vi "Intake And Elevator Loop.vi"(7 "Climbing?":bool) -> (3 "Intake Left Power":dbl, 4 "Intake Right Power":dbl, 6 "Intake Open":bool, 8 "Shift?":bool, 10 "Intake Angle":dbl, 15 "Elevator Power":dbl)   [LabVIEW 2017]
uses:
  Common Code/Intake And Elevator States.ctl
  Robot Global Data.vi
  <vilib>/addons/control/pid/pid.llb/PID (DBL).vi
  <vilib>/addons/control/pid/NI_PID_pid.lvlib
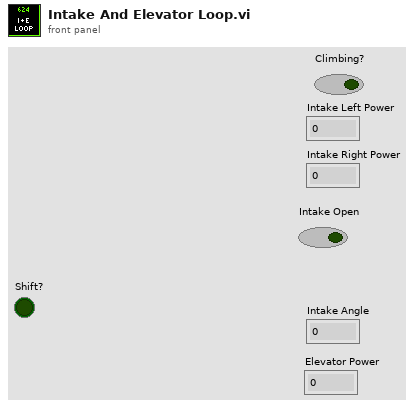
[diagram p1: front panel]
types:
  T1 = typedef "Intake And Elevator States.ctl" = enum16{"Reset", "Shoot Cube", "Drop Cube", "Idle", "Pick Up Cube", "Switch", "Scale ", "Endgame"}
  T2 = typedef "Intake And Elevator Command Cluster.ctl" = cluster{"States ":T1, "Grab?":bool, "Drop?":bool, "Mode":T3, "Override Lift":bool, "Override Lift":dbl, "High?":bool, "Override Angle":bool, "Override Angle":dbl}
  T3 = typedef "Intake and Elevator Mode.ctl" = enum16{"Auto", "Not Auto"}
  T4 = typedef "Dashboard Control Data.ctl" = cluster{"Drivetrain Settings Cluster":T5, "Intake Presets":T8, "Elevator Settings Cluster":T9, "Drivetrain Encoder Values":T11, "Auton Chooser":T12, "Auton Presets":cluster{"Start Position":dbl}, "Elevator Encoder Values":T13, "Pressure M":dbl, "Pressure B":dbl, "Zero All?":bool, "Enable Vision":bool}
  T5 = typedef "Drivetrain Settings Cluster.ctl" = cluster{"Gyro Steer PID Gains":T6, "Distance Drive PID Gains":T6, "Drive Tolerance":dbl, "Gyro Tolerance":dbl, "Gyro Output":dbl, "Distance Output":dbl, "Y Power Multiplier":dbl, "Turn Power Multiplier":dbl, "Creep Rate":dbl, "Encoder Reset":bool, "DT Mode Modifier":enum16{"None, Default", "Cube", "Square"}, "Left Encoder Tick Constant":dbl, "Right Encoder Tick Constant":dbl, "Shift Speed":dbl, "Zero Gyro":bool, "Y min":dbl, "Y max":dbl, "X min":dbl, "X max":dbl, "Finish Velocity":dbl, "Anti-Tip Settings":T7}
  T6 = typedef "PID Gains Cluster.ctl" = cluster{"Proportional Gain":dbl, "Integral Time":dbl, "Derivative Time":dbl}
  T7 = typedef "Anti-Tip Settings.ctl" = cluster{"Pitch Tip Constant":dbl, "Wheel Diameter":dbl, "Gearbox Reduction":dbl, "Motor Count":dbl, "Mass of Robot":dbl, "Almost Tip Constant":dbl, "Dist to CG":dbl}
  T8 = typedef "Intake Presets.ctl" = cluster{"Idle Angle":dbl, "Mid Angle":dbl, "Low Angle":dbl, "Outtake Power":dbl, "Intake Power":dbl, "Unstuck":dbl, "Angle Tolerance":dbl, "Max Angle":dbl, "Max Current":dbl, "Current Trip Time":dbl, "Reset Encoder?":bool, "Encoder Scale":dbl, "PID gains":cluster{"proportional gain (Kc)":dbl, "integral time (Ti, min)":dbl, "derivative time (Td, min)":dbl}, "output range":cluster{"output high":dbl, "output low":dbl}, "IR Constant Pull Rate":dbl, "Shoot Angle":dbl}
  T9 = typedef "Elevator Settings Cluster.ctl" = cluster{"Ground Height":dbl, "Switch Height":dbl, "Scale High Height ":dbl, "Scale Low Height":dbl, "Elevator PID Gains":T10, "Elevator Tolerance":dbl, "Reset Encoders":bool, "Encoder Scale":dbl, "Max Height":dbl, "Mid Height":dbl, "output range":cluster{"output high":dbl, "output low":dbl}, "Upper Slow Down Tolerance":dbl, "Tick Constant":dbl, "Tip Constant":dbl, "Slow Down Multiplier":dbl, "Almost Tip Constant":dbl, "Bottom Trip Offset":dbl, "Lower Slow Down Tolerance":dbl}
  T10 = typedef "PID Gains.ctl" = cluster{"proportional gain (Kc)":dbl, "integral time (Ti, min)":dbl, "derivative time (Td, min)":dbl}
  T11 = typedef "DT Encoder Values.ctl" = cluster{"Left Encoder":cluster{"Distance":dbl, "Speed":dbl, "Tick":dbl}, "Right Encoder":cluster{"Distance":dbl, "Speed":dbl, "Tick":dbl}}
  T12 = typedef "Auton Chooser.ctl" = cluster{"Left":bool, "Center":bool, "Right":bool, "Scale":bool, "Both":bool, "Switch":bool, "Test":bool, "No Script":bool, "Drive PID":bool, "Elevator PID":bool, "Gyro PID":bool}
  T13 = typedef "Elevator Encoder Values.ctl" = cluster{"Encoder Values":cluster{"Distance":dbl, "Speed":dbl, "Tick":dbl}}
  T14 = typedef "Elevator Status Cluster.ctl" = cluster{"Finished":bool, "Elevator Power":dbl, "Elevator State":T15, "Elevator Mode":T16, "Elevator Height":dbl, "At Bottom?":bool, "At Top?":bool, "Scale high?":bool, "PID Output":dbl, "2nd Gear":bool}
  T15 = typedef "Elevator State.ctl" = enum16{"Idle", "Ground", "Mid", "Scale", "Switch"}
  T16 = typedef "Elevator Mode.ctl" = enum16{"Semi Auto", "Manual", "Auto"}
  T17 = typedef "Intake Status Cluster.ctl" = cluster{"Intake Mode":T18, "Intake States":T19, "Intake Current Angle":dbl, "Cube In Posession?":bool, "Intake Wrist Up?":bool, "Right Roller Power":dbl, "Angle Power":dbl, "Left Roller Power":dbl}
  T18 = typedef "Intake Mode.ctl" = enum16{"Auto", "Semi Auto", "Manual"}
  T19 = typedef "Intake States.ctl" = enum16{"Zero", "Override Angle", "Idle", "Drop Mid", "Drop Low", "Outtake", "Intake"}
  T20 = cluster{"proportional gain (Kc)":dbl, "integral time (Ti, min)":dbl, "derivative time (Td, min)":dbl}
  T21 = typedef "Robot Info.ctl" = cluster{"FMS":bool, "Switch and Scale Sides":string, "Event Name":string, "Alliance":T22, "Position":T23, "Match Number":u16, "Robot Mode":T24, "Match Time(s)":sgl}
  T22 = typedef "WPI_DriverStationAllianceInfo.ctl" = enum16{"Red", "Blue", "Invalid"}
  T23 = typedef "WPI_DriverStationPositionInfo.ctl" = enum16{"1", "2", "3"}
  T24 = typedef "WPI_DriverStationRobotMode2.ctl" = enum16{"Autonomous Disabled", "Autonomous Enabled", "Teleop Disabled", "Teleop Enabled", "Disconnected", "Finish", "Test Disabled", "Test Enabled", "Emergency Stopped"}
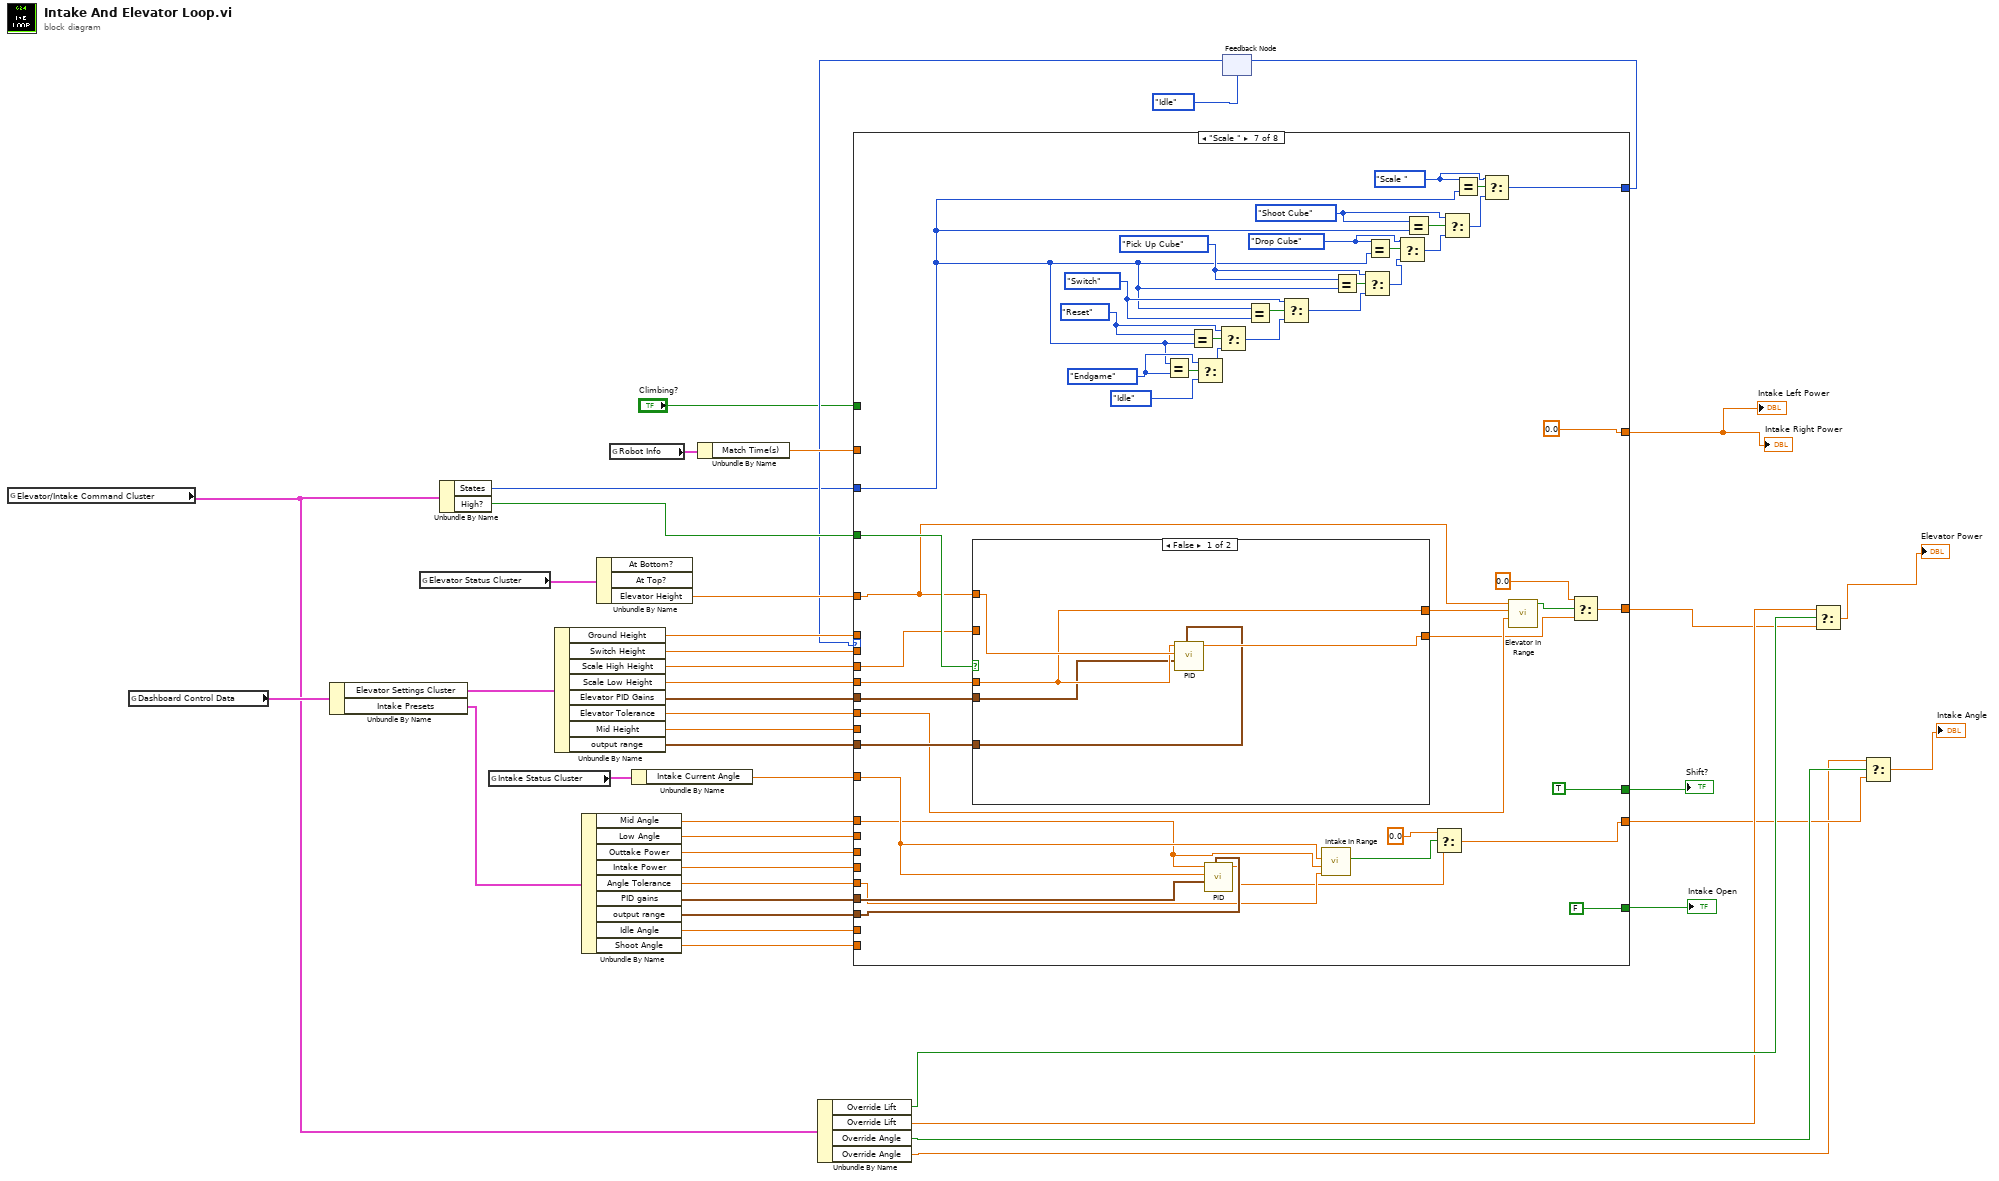
[diagram p0: block diagram]
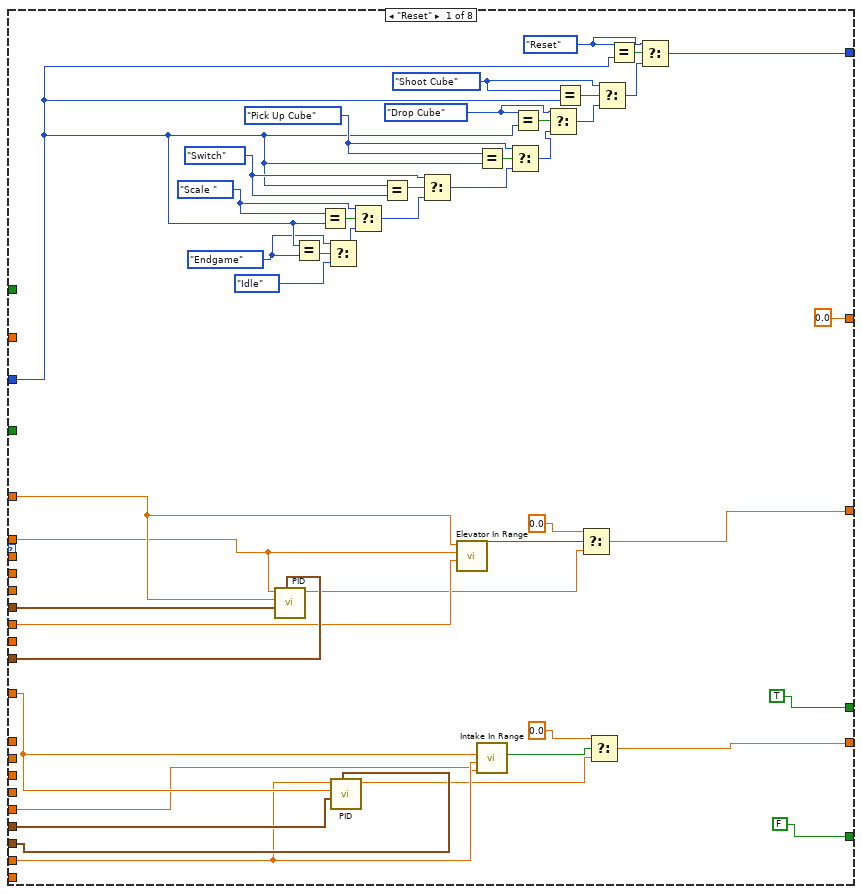
[diagram p2: hidden frame]
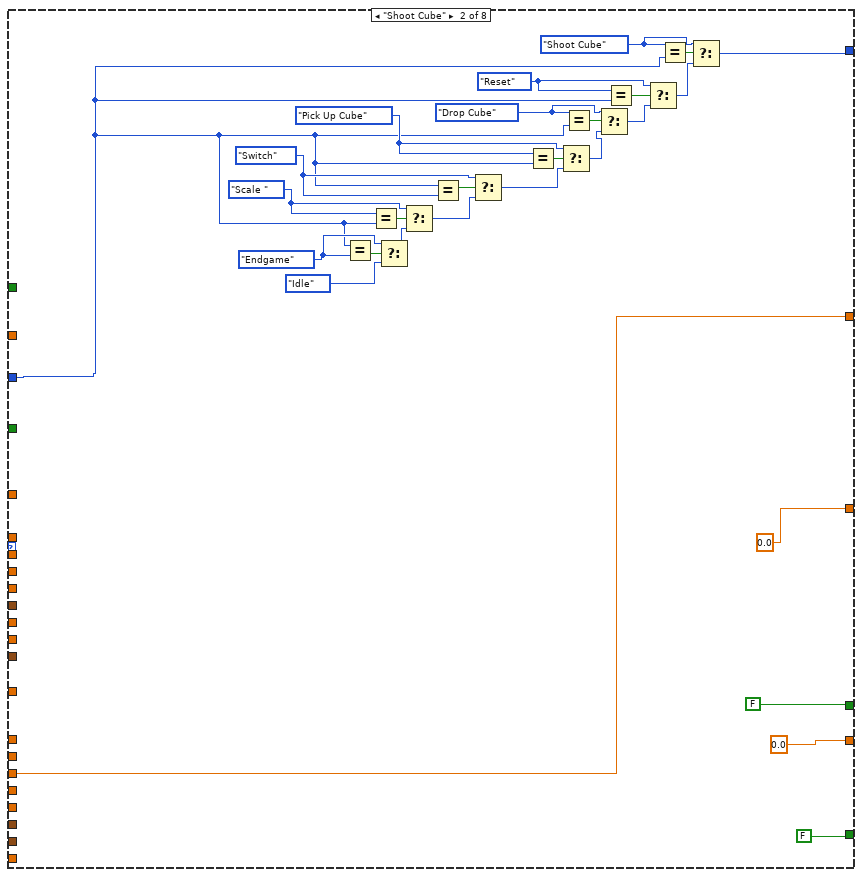
[diagram p3: hidden frame]
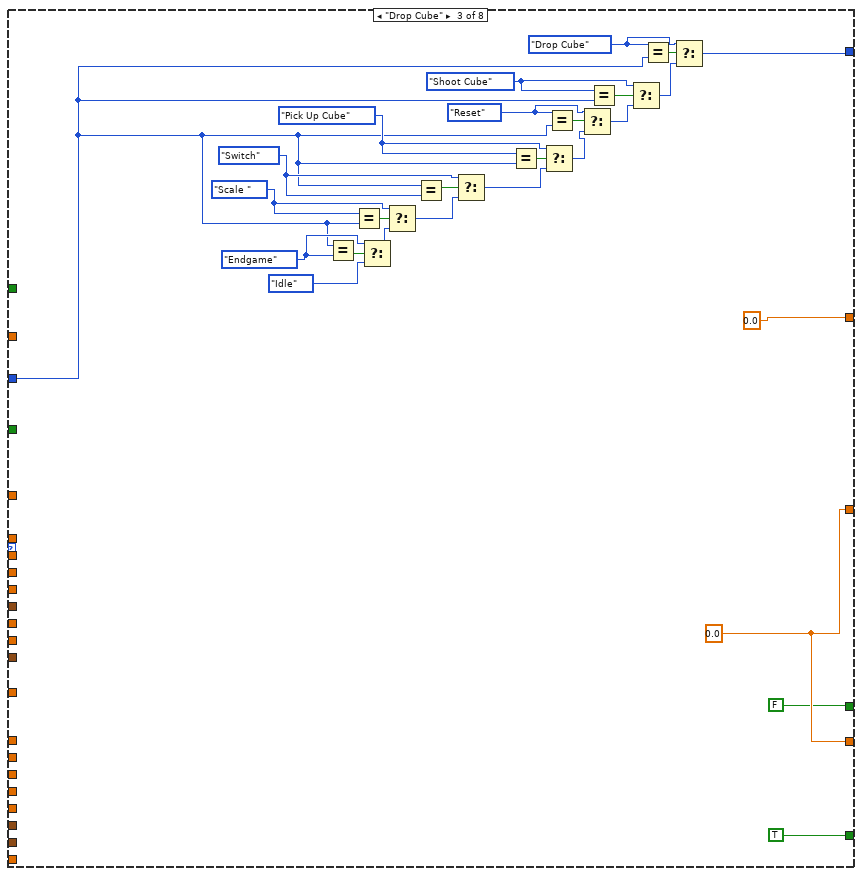
[diagram p4: hidden frame]
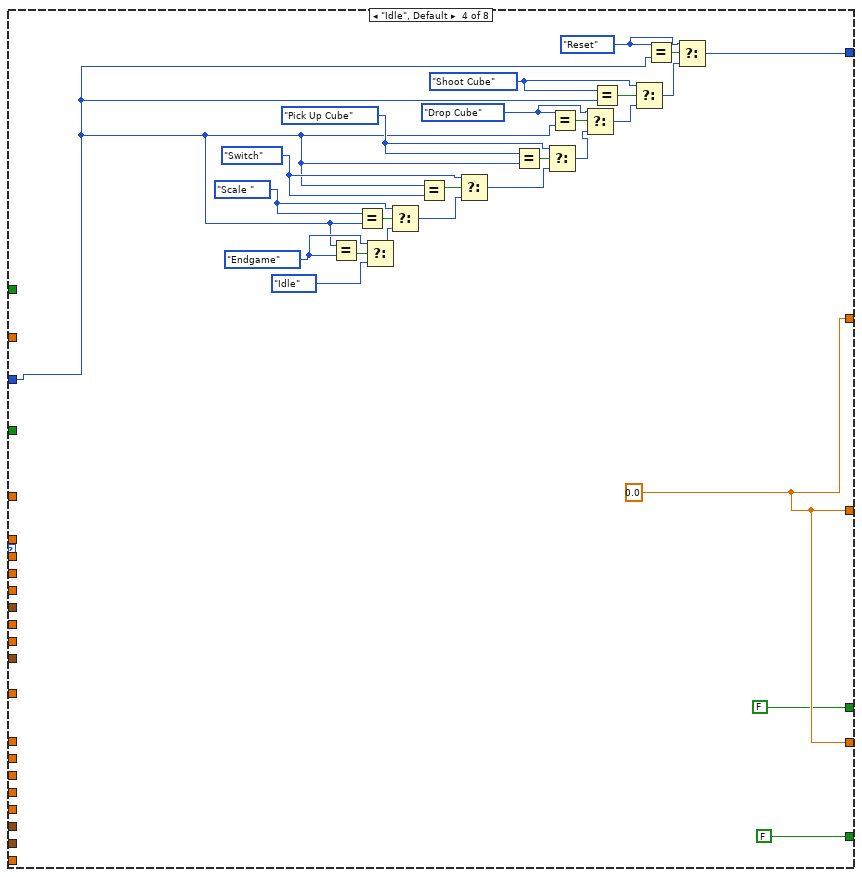
[diagram p5: hidden frame]
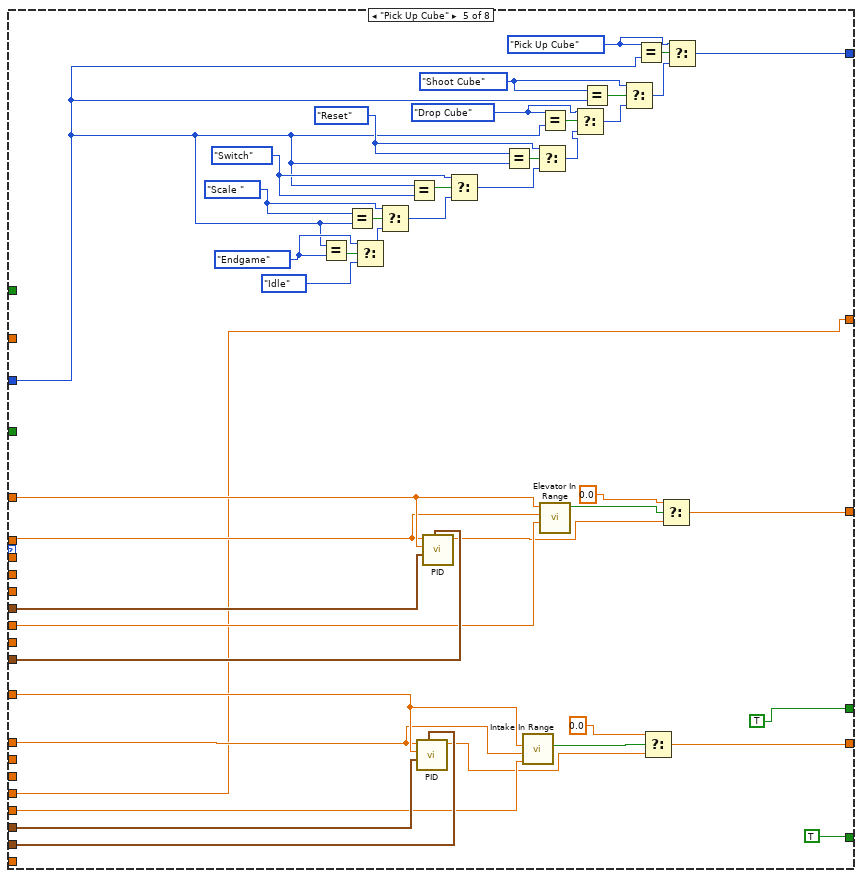
[diagram p6: hidden frame]
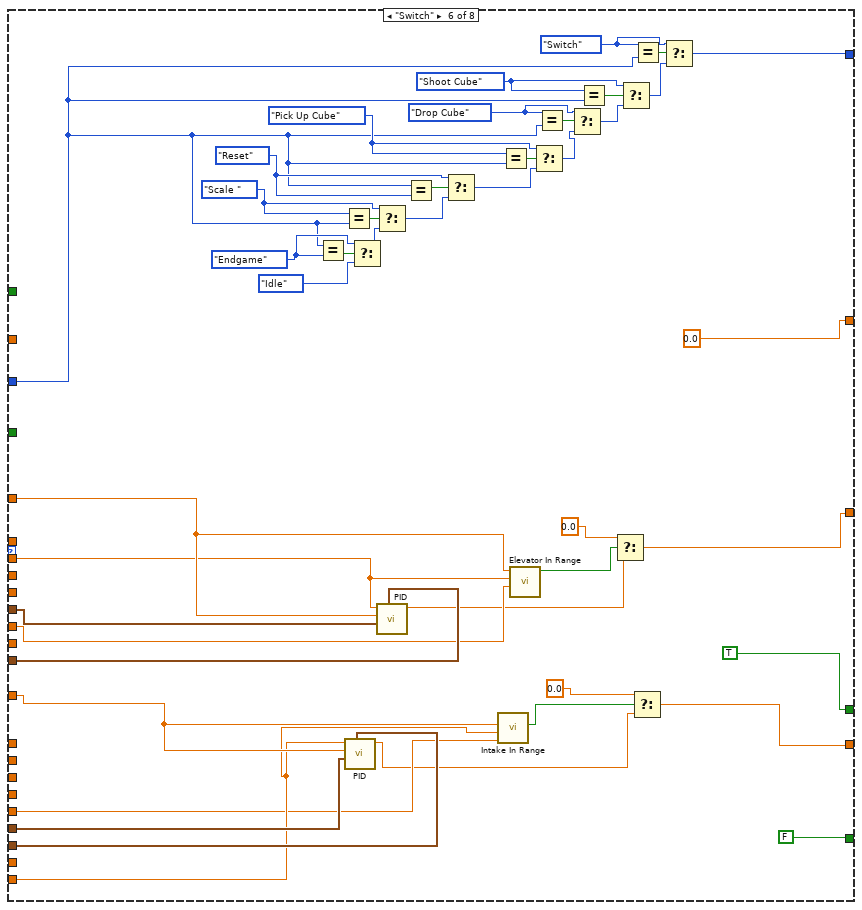
[diagram p7: hidden frame]
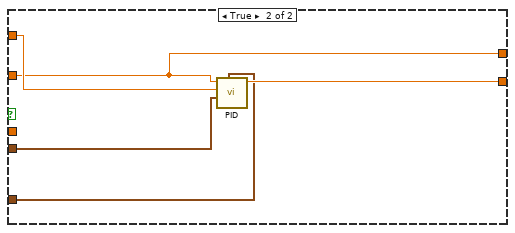
[diagram p8: hidden frame]
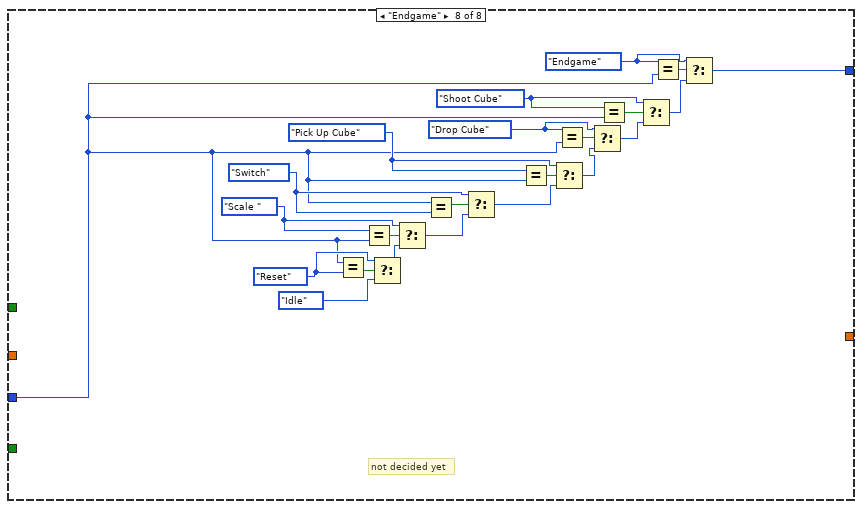
[diagram p9: hidden frame]
diagram:
  n1 = global read "Robot Global Data.vi" "Elevator/Intake Command Cluster"() -> (w9:T2)
  n2 = global read "Robot Global Data.vi" "Dashboard Control Data"() -> (w44:T4)
  n3 = Unbundle By Name(w44) -> ("Elevator Settings Cluster"=w43:T9, "Intake Presets"=w42:T8)
  n4 = global read "Robot Global Data.vi" "Elevator Status Cluster"() -> (w41:T14)
  n5 = Unbundle By Name(w9) -> ("States"=w12:T1, "High?"=w27:bool)
  n6 = global read "Robot Global Data.vi" "Intake Status Cluster"() -> (w40:T17)
  n7 = Unbundle By Name(w43) -> ("Ground Height"=w34:dbl, "Switch Height"=w28:dbl, "Scale High Height"=w26:dbl, "Scale Low Height"=w25:dbl, "Elevator PID Gains"=w32:T10, "Elevator Tolerance"=w30:dbl, "Mid Height"=w14:dbl, "output range"=w31:cluster{"output high":dbl, "output low":dbl})
  n8 = Unbundle By Name(w42) -> ("Mid Angle"=w29:dbl, "Low Angle"=w18:dbl, "Outtake Power"=w21:dbl, "Intake Power"=w19:dbl, "Angle Tolerance"=w37:dbl, "PID gains"=w35:T20, "output range"=w36:cluster{"output high":dbl, "output low":dbl}, "Idle Angle"=w39:dbl, "Shoot Angle"=w15:dbl)
  n9 = Unbundle By Name(w41) -> ("Elevator Height"=w33:dbl)  [unwired: 2 out]
  n10 = global read "Robot Global Data.vi" "Robot Info"() -> (w24:T21)
  n11 = Unbundle By Name(w40) -> ("Intake Current Angle"=w38:dbl)
  n12 = Unbundle By Name(w24) -> ("Match Time(s)"=w23:sgl)
  n13 = Unbundle By Name(w9) -> ("Override Lift"=w8:bool, "Override Lift"=w7:dbl, "Override Angle"=w4:bool, "Override Angle"=w1:dbl)
  n14 = feedback #1(Intake_And_Elevator_States."Idle" ("States")) -> (w13:T1)
  n15 = case shown="\"Scale \"" w13 {
    tunnel: w39 -> [w76 _ _ _ _ _ _ _]
    tunnel: w38 -> [w77 _ _ _ w203 w253 w290 _]
    tunnel: w37 -> [w75 _ _ _ w201 w251 w288 _]
    tunnel: w36 -> [w78 _ _ _ w212 w255 w291 _]
    tunnel: w35 -> [w79 _ _ _ w213 w254 w292 _]
    tunnel: w34 -> [w85 _ _ _ w208 _ _ _]
    tunnel: w33 -> [w86 _ _ _ w209 w246 w295 _]
    tunnel: w32 -> [w88 _ _ _ w211 w257 w301 _]
    tunnel: w31 -> [w87 _ _ _ w210 w256 w300 _]
    tunnel: w30 -> [w84 _ _ _ w207 w244 w297 _]
    tunnel: w29 -> [_ _ _ _ w202 _ w289 _]
    tunnel: w28 -> [_ _ _ _ _ w245 _ _]
    tunnel: w27 -> [_ _ _ _ _ _ w304 _]
    tunnel: w26 -> [_ _ _ _ _ _ w303 _]
    tunnel: w25 -> [_ _ _ _ _ _ w302 _]
    tunnel: w23 -> [_ _ _ _ _ _ _ _]
    tunnel: [w80 0.0 w142 w169 w197 w240 w299 _] -> w6
    tunnel: [w71 0.0 w142 w169 w196 w247 w284 _] -> w2
    tunnel: w21 -> [_ w114 _ _ _ _ _ _]
    tunnel: [0.0 w114 0.0 w169 w193 0.0 0.0 _] -> w20
    tunnel: w19 -> [_ _ _ _ w193 _ _ _]
    tunnel: w18 -> [_ _ _ _ _ _ _ _]
    tunnel: [FALSE FALSE TRUE FALSE TRUE FALSE FALSE _] -> w17
    tunnel: [TRUE FALSE FALSE FALSE TRUE TRUE TRUE _] -> w16
    tunnel: w15 -> [_ _ _ _ _ w252 _ _]
    tunnel: w14 -> [_ _ _ _ _ _ _ _]
    tunnel: w12 -> [w50 w90 w118 w145 w171 w215 w259 w316]
    tunnel: [w45 w89 w117 w144 w170 w214 w258 w315] -> w11
    tunnel: "Climbing?" -> [_ _ _ _ _ _ _ _]
    frame "Reset" {
      w48 = Intake_And_Elevator_States."Endgame" ("States")
      w52 = Intake_And_Elevator_States."Scale " ("States")
      w56 = Intake_And_Elevator_States."Switch" ("States")
      w58 = Intake_And_Elevator_States."Pick Up Cube" ("States")
      w61 = Intake_And_Elevator_States."Drop Cube" ("States")
      w64 = Intake_And_Elevator_States."Shoot Cube" ("States")
      w66 = Intake_And_Elevator_States."Reset" ("States")
      n16 = call-poly <vilib>:"PID.vi"("output range"=w87, "PID gains"=w88, "process variable"=w86, "setpoint"=w85) -> ("output"=w81:dbl)  [unwired: 6 in, 1 out]
      n17 = Equal?(x=w50, y=w48) -> (x = y?=w49:bool)
      n18 = Equal?(x=w52, y=w50) -> (x = y?=w53:bool)
      n19 = Select(t=w48, s=w49, f=Intake_And_Elevator_States."Idle" ("States")) -> (s? t:f=w47:T1)
      n20 = call-poly <vilib>:"PID.vi"("output range"=w78, "PID gains"=w79, "process variable"=w77, "setpoint"=w76) -> ("output"=w72:dbl)  [unwired: 6 in, 1 out]
      n21 = Select(t=w52, s=w53, f=w47) -> (s? t:f=w51:T1)
      n22 = Equal?(x=w50, y=w56) -> (x = y?=w57:bool)
      n23 = Select(t=w56, s=w57, f=w51) -> (s? t:f=w55:T1)
      n24 = call "Elevator In Range.vi"("Height Tolerance"=w84, "Target Height"=w85, "Actual Height"=w86) -> ("In Range"=w83:bool)  [unwired: 8 in]
      n25 = Equal?(x=w58, y=w50) -> (x = y?=w59:bool)
      n26 = call "Intake In Range.vi"("Angle Tolerance"=w75, "Target Height"=w76, "Actual Height"=w77) -> ("In Range?"=w74:bool)  [unwired: 8 in]
      n27 = Select(t=w58, s=w59, f=w55) -> (s? t:f=w54:T1)
      n28 = Equal?(x=w61, y=w50) -> (x = y?=w62:bool)
      n29 = Select(t=w61, s=w62, f=w54) -> (s? t:f=w60:T1)
      n30 = Equal?(x=w64, y=w50) -> (x = y?=w65:bool)
      n31 = Select(t=0.0, s=w83, f=w81) -> (s? t:f=w80:dbl)
      n32 = Select(t=0.0, s=w74, f=w72) -> (s? t:f=w71:dbl)
      n33 = Select(t=w64, s=w65, f=w60) -> (s? t:f=w63:T1)
      n34 = Equal?(x=w66, y=w50) -> (x = y?=w67:bool)
      n35 = Select(t=w66, s=w67, f=w63) -> (s? t:f=w45:T1)
    }
    frame "Shoot Cube" {
      w93 = Intake_And_Elevator_States."Endgame" ("States")
      w96 = Intake_And_Elevator_States."Scale " ("States")
      w100 = Intake_And_Elevator_States."Switch" ("States")
      w102 = Intake_And_Elevator_States."Pick Up Cube" ("States")
      w105 = Intake_And_Elevator_States."Drop Cube" ("States")
      w108 = Intake_And_Elevator_States."Reset" ("States")
      w110 = Intake_And_Elevator_States."Shoot Cube" ("States")
      n36 = Equal?(x=w90, y=w93) -> (x = y?=w94:bool)
      n37 = Equal?(x=w96, y=w90) -> (x = y?=w97:bool)
      n38 = Select(t=w93, s=w94, f=Intake_And_Elevator_States."Idle" ("States")) -> (s? t:f=w92:T1)
      n39 = Select(t=w96, s=w97, f=w92) -> (s? t:f=w95:T1)
      n40 = Equal?(x=w90, y=w100) -> (x = y?=w101:bool)
      n41 = Select(t=w100, s=w101, f=w95) -> (s? t:f=w99:T1)
      n42 = Equal?(x=w102, y=w90) -> (x = y?=w103:bool)
      n43 = Select(t=w102, s=w103, f=w99) -> (s? t:f=w98:T1)
      n44 = Equal?(x=w105, y=w90) -> (x = y?=w106:bool)
      n45 = Select(t=w105, s=w106, f=w98) -> (s? t:f=w104:T1)
      n46 = Equal?(x=w108, y=w90) -> (x = y?=w109:bool)
      n47 = Select(t=w108, s=w109, f=w104) -> (s? t:f=w107:T1)
      n48 = Equal?(x=w110, y=w90) -> (x = y?=w111:bool)
      n49 = Select(t=w110, s=w111, f=w107) -> (s? t:f=w89:T1)
    }
    frame "Drop Cube" {
      w121 = Intake_And_Elevator_States."Endgame" ("States")
      w124 = Intake_And_Elevator_States."Scale " ("States")
      w128 = Intake_And_Elevator_States."Switch" ("States")
      w130 = Intake_And_Elevator_States."Pick Up Cube" ("States")
      w133 = Intake_And_Elevator_States."Reset" ("States")
      w136 = Intake_And_Elevator_States."Shoot Cube" ("States")
      w138 = Intake_And_Elevator_States."Drop Cube" ("States")
      w142 = 0.0
      n50 = Equal?(x=w118, y=w121) -> (x = y?=w122:bool)
      n51 = Equal?(x=w124, y=w118) -> (x = y?=w125:bool)
      n52 = Select(t=w121, s=w122, f=Intake_And_Elevator_States."Idle" ("States")) -> (s? t:f=w120:T1)
      n53 = Select(t=w124, s=w125, f=w120) -> (s? t:f=w123:T1)
      n54 = Equal?(x=w118, y=w128) -> (x = y?=w129:bool)
      n55 = Select(t=w128, s=w129, f=w123) -> (s? t:f=w127:T1)
      n56 = Equal?(x=w130, y=w118) -> (x = y?=w131:bool)
      n57 = Select(t=w130, s=w131, f=w127) -> (s? t:f=w126:T1)
      n58 = Equal?(x=w133, y=w118) -> (x = y?=w134:bool)
      n59 = Select(t=w133, s=w134, f=w126) -> (s? t:f=w132:T1)
      n60 = Equal?(x=w136, y=w118) -> (x = y?=w137:bool)
      n61 = Select(t=w136, s=w137, f=w132) -> (s? t:f=w135:T1)
      n62 = Equal?(x=w138, y=w118) -> (x = y?=w139:bool)
      n63 = Select(t=w138, s=w139, f=w135) -> (s? t:f=w117:T1)
    }
    frame "Idle", Default {
      w148 = Intake_And_Elevator_States."Endgame" ("States")
      w151 = Intake_And_Elevator_States."Scale " ("States")
      w155 = Intake_And_Elevator_States."Switch" ("States")
      w157 = Intake_And_Elevator_States."Pick Up Cube" ("States")
      w160 = Intake_And_Elevator_States."Drop Cube" ("States")
      w163 = Intake_And_Elevator_States."Shoot Cube" ("States")
      w165 = Intake_And_Elevator_States."Reset" ("States")
      w169 = 0.0
      n64 = Equal?(x=w145, y=w148) -> (x = y?=w149:bool)
      n65 = Equal?(x=w151, y=w145) -> (x = y?=w152:bool)
      n66 = Select(t=w148, s=w149, f=Intake_And_Elevator_States."Idle" ("States")) -> (s? t:f=w147:T1)
      n67 = Select(t=w151, s=w152, f=w147) -> (s? t:f=w150:T1)
      n68 = Equal?(x=w145, y=w155) -> (x = y?=w156:bool)
      n69 = Select(t=w155, s=w156, f=w150) -> (s? t:f=w154:T1)
      n70 = Equal?(x=w157, y=w145) -> (x = y?=w158:bool)
      n71 = Select(t=w157, s=w158, f=w154) -> (s? t:f=w153:T1)
      n72 = Equal?(x=w160, y=w145) -> (x = y?=w161:bool)
      n73 = Select(t=w160, s=w161, f=w153) -> (s? t:f=w159:T1)
      n74 = Equal?(x=w163, y=w145) -> (x = y?=w164:bool)
      n75 = Select(t=w163, s=w164, f=w159) -> (s? t:f=w162:T1)
      n76 = Equal?(x=w165, y=w145) -> (x = y?=w166:bool)
      n77 = Select(t=w165, s=w166, f=w162) -> (s? t:f=w144:T1)
    }
    frame "Pick Up Cube" {
      w174 = Intake_And_Elevator_States."Endgame" ("States")
      w177 = Intake_And_Elevator_States."Scale " ("States")
      w181 = Intake_And_Elevator_States."Switch" ("States")
      w183 = Intake_And_Elevator_States."Reset" ("States")
      w186 = Intake_And_Elevator_States."Drop Cube" ("States")
      w189 = Intake_And_Elevator_States."Shoot Cube" ("States")
      w191 = Intake_And_Elevator_States."Pick Up Cube" ("States")
      n78 = Equal?(x=w171, y=w174) -> (x = y?=w175:bool)
      n79 = Equal?(x=w177, y=w171) -> (x = y?=w178:bool)
      n80 = Select(t=w174, s=w175, f=Intake_And_Elevator_States."Idle" ("States")) -> (s? t:f=w173:T1)
      n81 = Select(t=w177, s=w178, f=w173) -> (s? t:f=w176:T1)
      n82 = Equal?(x=w171, y=w181) -> (x = y?=w182:bool)
      n83 = call-poly <vilib>:"PID.vi"("output range"=w212, "PID gains"=w213, "process variable"=w203, "setpoint"=w202) -> ("output"=w198:dbl)  [unwired: 6 in, 1 out]
      n84 = call-poly <vilib>:"PID.vi"("output range"=w210, "PID gains"=w211, "process variable"=w209, "setpoint"=w208) -> ("output"=w204:dbl)  [unwired: 6 in, 1 out]
      n85 = Select(t=w181, s=w182, f=w176) -> (s? t:f=w180:T1)
      n86 = Equal?(x=w183, y=w171) -> (x = y?=w184:bool)
      n87 = call "Intake In Range.vi"("Angle Tolerance"=w201, "Target Height"=w202, "Actual Height"=w203) -> ("In Range?"=w200:bool)  [unwired: 8 in]
      n88 = Select(t=w183, s=w184, f=w180) -> (s? t:f=w179:T1)
      n89 = Equal?(x=w186, y=w171) -> (x = y?=w187:bool)
      n90 = call "Elevator In Range.vi"("Height Tolerance"=w207, "Target Height"=w208, "Actual Height"=w209) -> ("In Range"=w206:bool)  [unwired: 8 in]
      n91 = Select(t=w186, s=w187, f=w179) -> (s? t:f=w185:T1)
      n92 = Equal?(x=w189, y=w171) -> (x = y?=w190:bool)
      n93 = Select(t=w189, s=w190, f=w185) -> (s? t:f=w188:T1)
      n94 = Equal?(x=w191, y=w171) -> (x = y?=w192:bool)
      n95 = Select(t=0.0, s=w200, f=w198) -> (s? t:f=w196:dbl)
      n96 = Select(t=0.0, s=w206, f=w204) -> (s? t:f=w197:dbl)
      n97 = Select(t=w191, s=w192, f=w188) -> (s? t:f=w170:T1)
    }
    frame "Switch" {
      w218 = Intake_And_Elevator_States."Endgame" ("States")
      w221 = Intake_And_Elevator_States."Scale " ("States")
      w225 = Intake_And_Elevator_States."Reset" ("States")
      w227 = Intake_And_Elevator_States."Pick Up Cube" ("States")
      w230 = Intake_And_Elevator_States."Drop Cube" ("States")
      w233 = Intake_And_Elevator_States."Shoot Cube" ("States")
      w235 = Intake_And_Elevator_States."Switch" ("States")
      n98 = Equal?(x=w215, y=w218) -> (x = y?=w219:bool)
      n99 = Equal?(x=w221, y=w215) -> (x = y?=w222:bool)
      n100 = call-poly <vilib>:"PID.vi"("output range"=w255, "PID gains"=w254, "process variable"=w253, "setpoint"=w252) -> ("output"=w248:dbl)  [unwired: 6 in, 1 out]
      n101 = Select(t=w218, s=w219, f=Intake_And_Elevator_States."Idle" ("States")) -> (s? t:f=w217:T1)
      n102 = Select(t=w221, s=w222, f=w217) -> (s? t:f=w220:T1)
      n103 = call-poly <vilib>:"PID.vi"("output range"=w256, "PID gains"=w257, "process variable"=w246, "setpoint"=w245) -> ("output"=w241:dbl)  [unwired: 6 in, 1 out]
      n104 = Equal?(x=w215, y=w225) -> (x = y?=w226:bool)
      n105 = Select(t=w225, s=w226, f=w220) -> (s? t:f=w224:T1)
      n106 = call "Intake In Range.vi"("Angle Tolerance"=w251, "Target Height"=w252, "Actual Height"=w253) -> ("In Range?"=w250:bool)  [unwired: 8 in]
      n107 = Equal?(x=w227, y=w215) -> (x = y?=w228:bool)
      n108 = call "Elevator In Range.vi"("Height Tolerance"=w244, "Target Height"=w245, "Actual Height"=w246) -> ("In Range"=w243:bool)  [unwired: 8 in]
      n109 = Select(t=w227, s=w228, f=w224) -> (s? t:f=w223:T1)
      n110 = Equal?(x=w230, y=w215) -> (x = y?=w231:bool)
      n111 = Select(t=w230, s=w231, f=w223) -> (s? t:f=w229:T1)
      n112 = Equal?(x=w233, y=w215) -> (x = y?=w234:bool)
      n113 = Select(t=0.0, s=w243, f=w241) -> (s? t:f=w240:dbl)
      n114 = Select(t=w233, s=w234, f=w229) -> (s? t:f=w232:T1)
      n115 = Select(t=0.0, s=w250, f=w248) -> (s? t:f=w247:dbl)
      n116 = Equal?(x=w235, y=w215) -> (x = y?=w236:bool)
      n117 = Select(t=w235, s=w236, f=w232) -> (s? t:f=w214:T1)
    }
    frame "Scale " {
      w262 = Intake_And_Elevator_States."Endgame" ("States")
      w265 = Intake_And_Elevator_States."Reset" ("States")
      w269 = Intake_And_Elevator_States."Switch" ("States")
      w271 = Intake_And_Elevator_States."Pick Up Cube" ("States")
      w274 = Intake_And_Elevator_States."Drop Cube" ("States")
      w277 = Intake_And_Elevator_States."Shoot Cube" ("States")
      w279 = Intake_And_Elevator_States."Scale " ("States")
      n118 = case shown="False" w304 {
        tunnel: w303 -> [_ w310]
        tunnel: w302 -> [w308 _]
        tunnel: w301 -> [w305 w312]
        tunnel: w300 -> [w306 w311]
        tunnel: [w307 w314] -> w294
        tunnel: [w308 w310] -> w296
        tunnel: w295 -> [w309 w313]
        frame False {
          n119 = call-poly <vilib>:"PID.vi"("output range"=w306, "PID gains"=w305, "process variable"=w309, "setpoint"=w308) -> ("output"=w307:dbl)  [unwired: 6 in, 1 out]
        }
        frame True {
          n120 = call-poly <vilib>:"PID.vi"("output range"=w311, "PID gains"=w312, "process variable"=w313, "setpoint"=w310) -> ("output"=w314:dbl)  [unwired: 6 in, 1 out]
        }
      }
      n121 = Equal?(x=w259, y=w262) -> (x = y?=w263:bool)
      n122 = Equal?(x=w265, y=w259) -> (x = y?=w266:bool)
      n123 = Select(t=w262, s=w263, f=Intake_And_Elevator_States."Idle" ("States")) -> (s? t:f=w261:T1)
      n124 = call-poly <vilib>:"PID.vi"("output range"=w291, "PID gains"=w292, "process variable"=w290, "setpoint"=w289) -> ("output"=w286:dbl)  [unwired: 6 in, 1 out]
      n125 = Select(t=w265, s=w266, f=w261) -> (s? t:f=w264:T1)
      n126 = Equal?(x=w259, y=w269) -> (x = y?=w270:bool)
      n127 = Select(t=w269, s=w270, f=w264) -> (s? t:f=w268:T1)
      n128 = call "Intake In Range.vi"("Angle Tolerance"=w288, "Target Height"=w289, "Actual Height"=w290) -> ("In Range?"=w287:bool)  [unwired: 8 in]
      n129 = Equal?(x=w271, y=w259) -> (x = y?=w272:bool)
      n130 = Select(t=w271, s=w272, f=w268) -> (s? t:f=w267:T1)
      n131 = Equal?(x=w274, y=w259) -> (x = y?=w275:bool)
      n132 = Select(t=w274, s=w275, f=w267) -> (s? t:f=w273:T1)
      n133 = Equal?(x=w277, y=w259) -> (x = y?=w278:bool)
      n134 = Select(t=0.0, s=w287, f=w286) -> (s? t:f=w284:dbl)
      n135 = Select(t=w277, s=w278, f=w273) -> (s? t:f=w276:T1)
      n136 = Equal?(x=w279, y=w259) -> (x = y?=w280:bool)
      n137 = Select(t=w279, s=w280, f=w276) -> (s? t:f=w258:T1)
      n138 = call "Elevator In Range.vi"("Height Tolerance"=w297, "Target Height"=w296, "Actual Height"=w295) -> ("In Range"=w298:bool)  [unwired: 8 in]
      n139 = Select(t=0.0, s=w298, f=w294) -> (s? t:f=w299:dbl)
    }
    frame "Endgame" {
      w319 = Intake_And_Elevator_States."Reset" ("States")
      w322 = Intake_And_Elevator_States."Scale " ("States")
      w326 = Intake_And_Elevator_States."Switch" ("States")
      w328 = Intake_And_Elevator_States."Pick Up Cube" ("States")
      w331 = Intake_And_Elevator_States."Drop Cube" ("States")
      w334 = Intake_And_Elevator_States."Shoot Cube" ("States")
      w336 = Intake_And_Elevator_States."Endgame" ("States")
      # "not decided yet"
      n140 = Equal?(x=w316, y=w319) -> (x = y?=w320:bool)
      n141 = Equal?(x=w322, y=w316) -> (x = y?=w323:bool)
      n142 = Select(t=w319, s=w320, f=Intake_And_Elevator_States."Idle" ("States")) -> (s? t:f=w318:T1)
      n143 = Select(t=w322, s=w323, f=w318) -> (s? t:f=w321:T1)
      n144 = Equal?(x=w316, y=w326) -> (x = y?=w327:bool)
      n145 = Select(t=w326, s=w327, f=w321) -> (s? t:f=w325:T1)
      n146 = Equal?(x=w328, y=w316) -> (x = y?=w329:bool)
      n147 = Select(t=w328, s=w329, f=w325) -> (s? t:f=w324:T1)
      n148 = Equal?(x=w331, y=w316) -> (x = y?=w332:bool)
      n149 = Select(t=w331, s=w332, f=w324) -> (s? t:f=w330:T1)
      n150 = Equal?(x=w334, y=w316) -> (x = y?=w335:bool)
      n151 = Select(t=w334, s=w335, f=w330) -> (s? t:f=w333:T1)
      n152 = Equal?(x=w336, y=w316) -> (x = y?=w337:bool)
      n153 = Select(t=w336, s=w337, f=w333) -> (s? t:f=w315:T1)
    }
  }
  "Intake Left Power" <- w20
  "Intake Right Power" <- w20
  "Intake Open" <- w17
  "Shift?" <- w16
  n154 = feedback-in #1(w11) -> ()
  n155 = Select(t=w7, s=w8, f=w6) -> (s? t:f=→"Elevator Power":dbl)
  n156 = Select(t=w1, s=w4, f=w2) -> (s? t:f=→"Intake Angle":dbl)
